vi "ParseFeedPackageMeta.vi"(8 "Error In":errorcluster, 10 "FeedURL":string, 11 "FeedPackageMeta":string) -> (0 "Error Out":errorcluster, 2 "PackageMetaMap":map{string, string}[](array[numeric]), 3 "PackageMeta":T1[](array[typedef]))   [LabVIEW 2019, in "CEPM.lvlib"]
uses:
  CEPM.lvlib
  Typedefs/PackageMeta.ctl
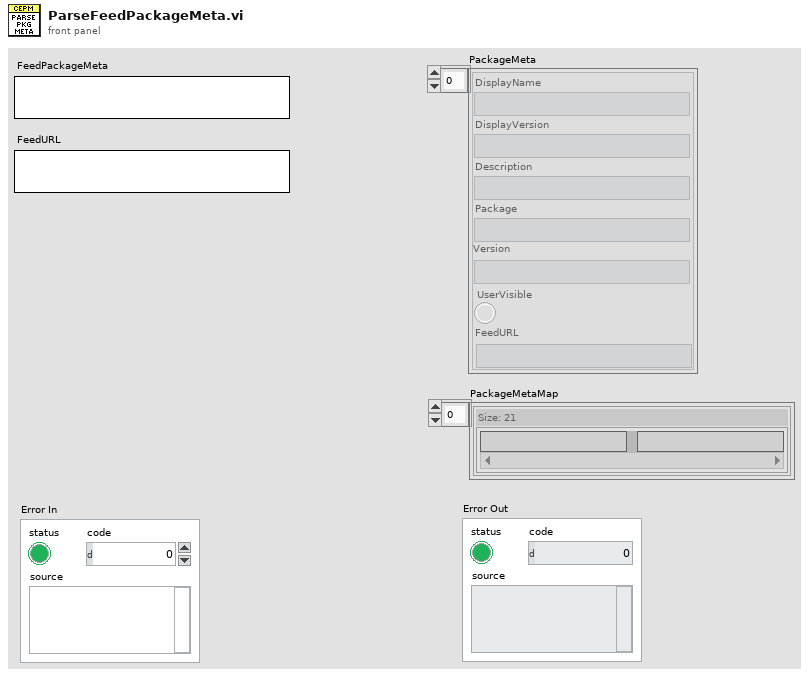
[diagram p1: front panel]
types:
  T1 = typedef "CEPM.lvlib/PackageMeta.ctl" = cluster{"DisplayName":string, "DisplayVersion":string, "Description":string, "Package":string, "Version":string, "UserVisible":bool, "FeedURL":string}
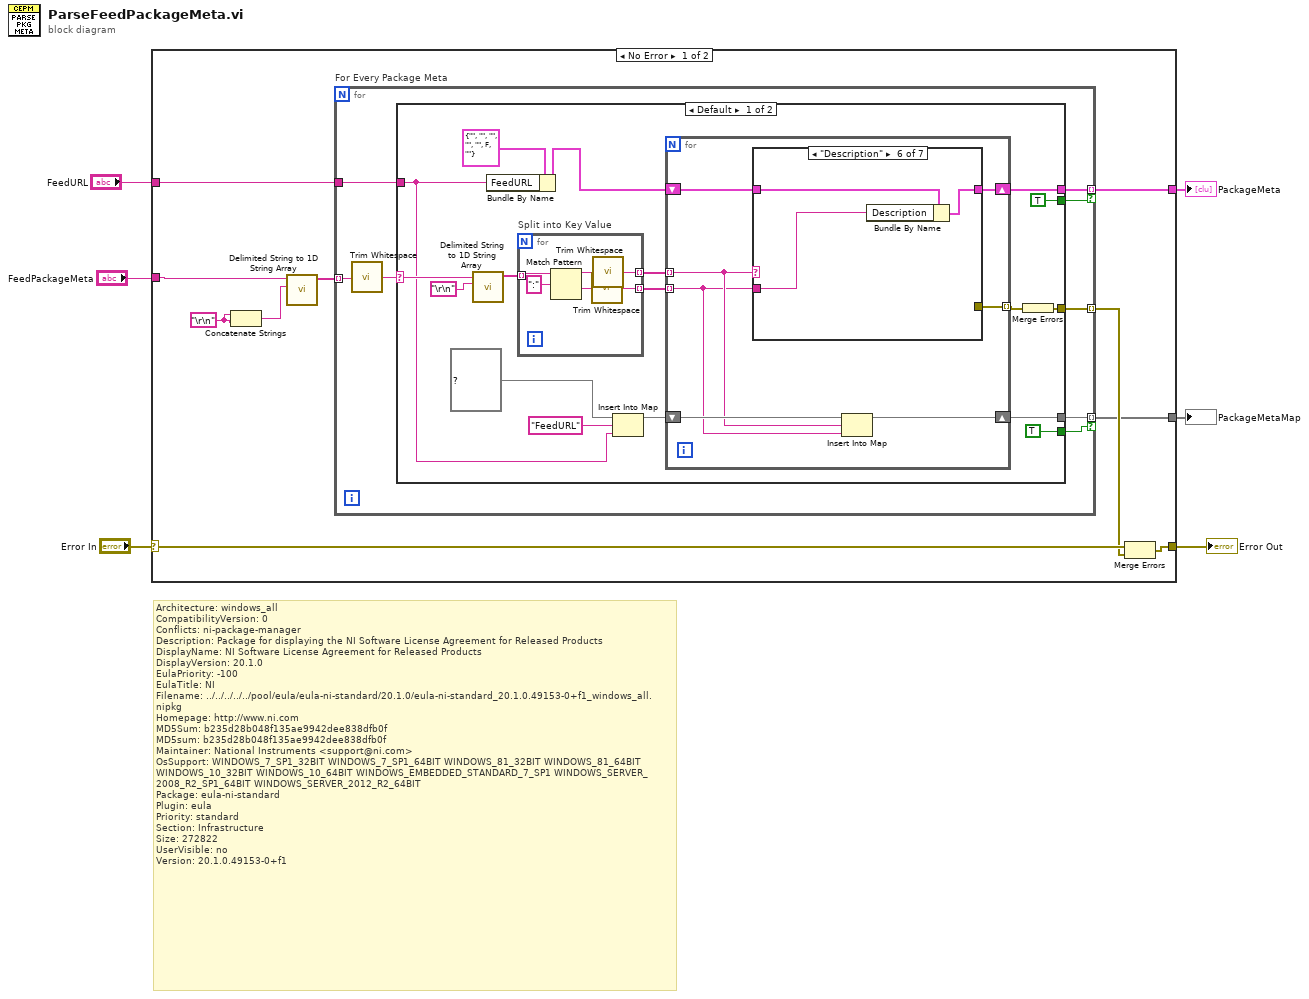
[diagram p0: block diagram]
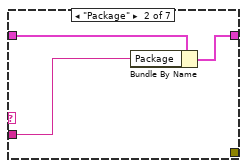
[diagram p3: hidden frame]
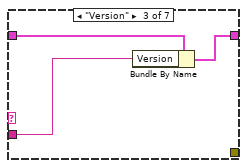
[diagram p4: hidden frame]
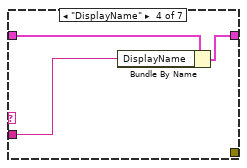
[diagram p5: hidden frame]
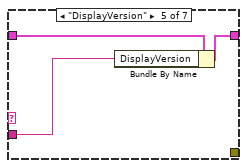
[diagram p6: hidden frame]
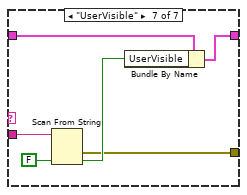
[diagram p7: hidden frame]
diagram:
  # "﻿Architecture: windows_all\nCompatibilityVersion: 0\nConflicts: ni-package-manager\nDescription: Package for displaying the NI Software License Agreement for Released Products\nDisplayName: NI Software License Agreement for Released Products\nDisplayVersion: 20.1.0\nEulaPriority: -100\nEulaTitle: NI\nFilename: ../../../../../pool/eula/eula-ni-standard/20.1.0/eula-ni-standard_20.1.0.49153-0+f1_windows_all.nipkg\nHomepage: http://www.ni.com\nMD5Sum: b235d28b048f135ae9942dee838dfb0f\nMD5sum: b235d28b048f135ae9942dee838dfb0f\nMaintainer: National Instruments <support@ni.com>\nOsSupport: WINDOWS_7_SP1_32BIT WINDOWS_7_SP1_64BIT WINDOWS_81_32BIT WINDOWS_81_64BIT WINDOWS_10_32BIT WINDOWS_10_64BIT WINDOWS_EMBEDDED_STANDARD_7_SP1 WINDOWS_SERVER_2008_R2_SP1_64BIT WINDOWS_SERVER_2012_R2_64BIT\nPackage: eula-ni-standard\nPlugin: eula\nPriority: standard\nSection: Infrastructure\nSize: 272822\nUserVisible: no\nVersion: 20.1.0.49153-0+f1"
  n1 = case shown="No Error" "Error In" {
    selector: "Error In" -> [w12 w77]
    tunnel: [w11 w77] -> w5
    tunnel: "FeedPackageMeta" -> [w14 _]
    tunnel: [w9 _] -> w3
    tunnel: [w8 _] -> w2
    tunnel: "FeedURL" -> [w7 _]
    frame No Error {
      w16 = "\r\n"
      n2 = Concatenate Strings(w16, w16) -> (w15:string)
      n3 = call <vilib>:"Delimited String to 1D String Array.vi"("delimiter"=w15, "delimited string"=w14) -> ("string array"=w13:string[])  [unwired: 9 in]
      n4 = for "For Every Package Meta" {
        tunnel: w13 -> [w24] mode=indexing
        tunnel: [w22] -> w10 mode=indexing
        tunnel: [w21] -> w9 mode=indexing if=w20
        tunnel: [w19] -> w8 mode=indexing if=w18
        tunnel: w7 -> [w17]
        n5 = call <vilib>:"Trim Whitespace.vi"("string"=w24) -> ("trimmed string"=w23:string)  [unwired: 1 in]
        n6 = case shown="Default" w23 {
          selector: w23 -> [w41 _]
          tunnel: [w34 _] -> w22
          tunnel: [w33 _] -> w21
          tunnel: [TRUE _] -> w20
          tunnel: [w31 _] -> w19
          tunnel: [TRUE _] -> w18
          tunnel: w17 -> [w25 _]
          frame Default {
            n7 = call <vilib>:"Delimited String to 1D String Array.vi"("delimiter"="\r\n", "delimited string"=w41) -> ("string array"=w39:string[])  [unwired: 9 in]
            n8 = Bundle By Name(cluster=T1 {"DisplayName"="", "DisplayVersion"="", "Description"="", "Package"="", "Version"="", "UserVisible"=FALSE, "FeedURL"=""} ("PackageMeta"), "FeedURL"=w25) -> (w29:T1)
            n9 = for "Split into Key Value" {
              tunnel: w39 -> [w76] mode=indexing
              tunnel: [w72] -> w38 mode=indexing
              tunnel: [w71] -> w37 mode=indexing
              n10 = Match Pattern(string=w76, regular expression=":") -> (before substring=w74:string, after substring=w73:string)  [unwired: 1 in, 2 out]
              n11 = call <vilib>:"Trim Whitespace.vi"("string"=w73) -> ("trimmed string"=w71:string)  [unwired: 1 in]
              n12 = call <vilib>:"Trim Whitespace.vi"("string"=w74) -> ("trimmed string"=w72:string)  [unwired: 1 in]
            }
            n13 = Insert Into Map(map in=map{string, string} {} ("map"), key="FeedURL", value=w25) -> (map out=w27:map{string, string})  [unwired: 2 out]
            n14 = for {
              tunnel: w38 -> [w44] mode=indexing
              tunnel: w37 -> [w43] mode=indexing
              shift-right: [w47] -> w33
              shift-left: w29 -> [w48]
              tunnel: [w46] -> w35 mode=indexing
              shift-right: [w42] -> w31
              shift-left: w27 -> [w45]
              n15 = case shown="\"Description\"" w44 {
                tunnel: w43 -> [_ w50 w53 w56 w59 w62 w68]
                tunnel: w48 -> [w49 w52 w55 w58 w61 w64 w70]
                tunnel: [w49 w51 w54 w57 w60 w63 w69] -> w47
                tunnel: [_ _ _ _ _ _ w65] -> w46
                frame Default {
                }
                frame "Package" {
                  n16 = Bundle By Name(cluster=w52, "Package"=w50) -> (w51:T1)
                }
                frame "Version" {
                  n17 = Bundle By Name(cluster=w55, "Version"=w53) -> (w54:T1)
                }
                frame "DisplayName" {
                  n18 = Bundle By Name(cluster=w58, "DisplayName"=w56) -> (w57:T1)
                }
                frame "DisplayVersion" {
                  n19 = Bundle By Name(cluster=w61, "DisplayVersion"=w59) -> (w60:T1)
                }
                frame "Description" {
                  n20 = Bundle By Name(cluster=w64, "Description"=w62) -> (w63:T1)
                }
                frame "UserVisible" {
                  n21 = Scan From String(input string=w68, default 1=FALSE) -> (error out=w65:errorcluster, output 1=w66:bool)  [unwired: 3 in, 2 out]
                  n22 = Bundle By Name(cluster=w70, "UserVisible"=w66) -> (w69:T1)
                }
              }
              n23 = Insert Into Map(map in=w45, key=w44, value=w43) -> (map out=w42:map{string, string})  [unwired: 2 out]
            }
            n24 = Merge Errors(w35) -> (w34:errorcluster)
          }
          frame "" {
          }
        }
      }
      n25 = Merge Errors(w12, w10) -> (w11:errorcluster)
    }
    frame Error {
    }
  }
  "Error Out" <- w5
  "PackageMeta" <- w3
  "PackageMetaMap" <- w2
